vi "thickness main.vi"() -> ()   [LabVIEW 2014]
uses:
  <vilib>/userdefined/High Color/IMAQdx.ctl
  <vilib>/vision/driver/NI_Vision_Acquisition_Software.lvlib
  <vilib>/vision/NI_Vision_Development_Module.lvlib
  <vilib>/Analysis/NI_AALBase.lvlib
  <vilib>/ptbypt/NI_PtbyPt.lvlib
panel:
  in  "탭 컨트롤":enum32{"두께 측정", "vision set", "공정능력"}(tab)
  in  "두께보정":sgl=0.008
  in  "측정속도(sec)":i8
  in  "Camera Name 2":T1="cam0"
  out "Image Out":T2(plugin-control)
  out "mm":sgl
  out "Image 2":T2(plugin-control)
  out "웨이브폼 차트 3":sgl(graph)
  in  "정지 3":bool
  out "Cpk":dbl(graph)
  in  "하한규격":dbl=1.7 format="%_3f"
  in  "상한규격":dbl=1.8 format="%_3f"
  in  "측정":T3={"Contrast"=1, "Filter width"=11, "Steepness"=0, "Subsampling Ratio"=100, "Show Search Area"=TRUE, "Show Search Lines"=TRUE, "Show Edges Found"=TRUE, "Show Result"=TRUE}
  in  "입자 수":i32=20
  in  "Blue or Luma or Val or Inten":cluster{"Lower value":i32, "Upper value":i32}={"Lower value"=0, "Upper value"=93}
  in  "Green or Sat":cluster{"Lower value":i32, "Upper value":i32}={"Lower value"=0, "Upper value"=179}
  in  "Red or Hue":cluster{"Lower value":i32, "Upper value":i32}={"Lower value"=0, "Upper value"=246}
  out "Image Out 2":T2(plugin-control)
  out "Histogram":T4(graph)
  out "mm":dbl
  in  "intervals":i32=20
  out "Cpk":dbl format="%#_3g"
  out "Minimum":dbl format="%_3g"
  out "Maximum":dbl format="%#_3g"
  out "Standard Dev":dbl format="%#_3g"
  out "mean":dbl format="%.3f"
  # "칼러필터"
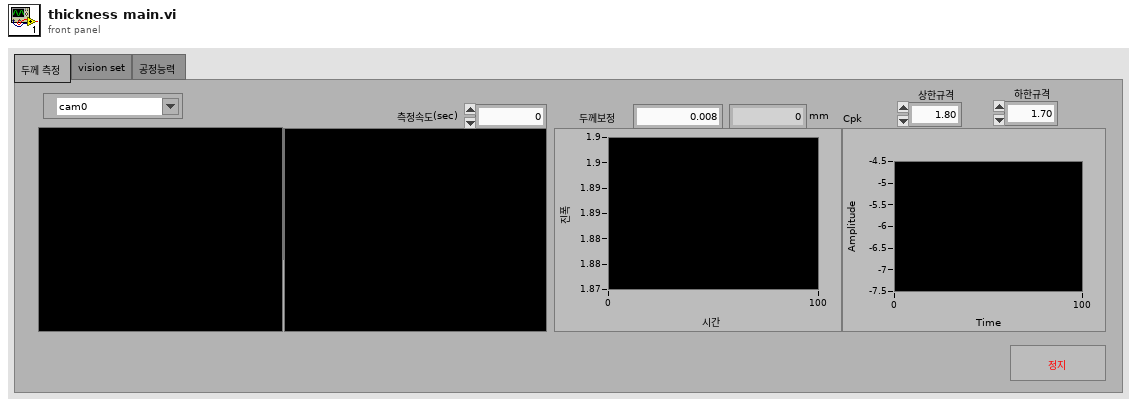
[diagram p1: front panel]
types:
  T1 = typedef "IMAQdx.ctl" = refnum<k21>
  T2 = typedef "IMAQ Image.ctl" = refnum<image>
  T3 = cluster{"Contrast":i32, "Filter width":i32, "Steepness":i32, "Subsampling Ratio":u32, "Show Search Area":bool, "Show Search Lines":bool, "Show Edges Found":bool, "Show Result":bool}
  T4 = cluster{"X Values":dbl[], "Histogram: h(x)":i32[]}
  T5 = cluster{"Global Rectangle":i32[], "Contours":cluster{"ID":enum32{"External", "Internal"}, "Type":u32, "Coordinates":i32[]}[]}
  T6 = cluster{"mm":sgl, "mm":sgl, "mm":sgl, "mm":sgl, "mm":sgl, "mm":sgl, "mm":sgl, "mm":sgl, "mm":sgl, "mm":sgl, "mm":sgl, "mm":sgl, "mm":sgl, "mm":sgl, "mm":sgl, "mm":sgl, "mm":sgl, "mm":sgl, "mm":sgl, "mm":sgl, "mm":sgl}
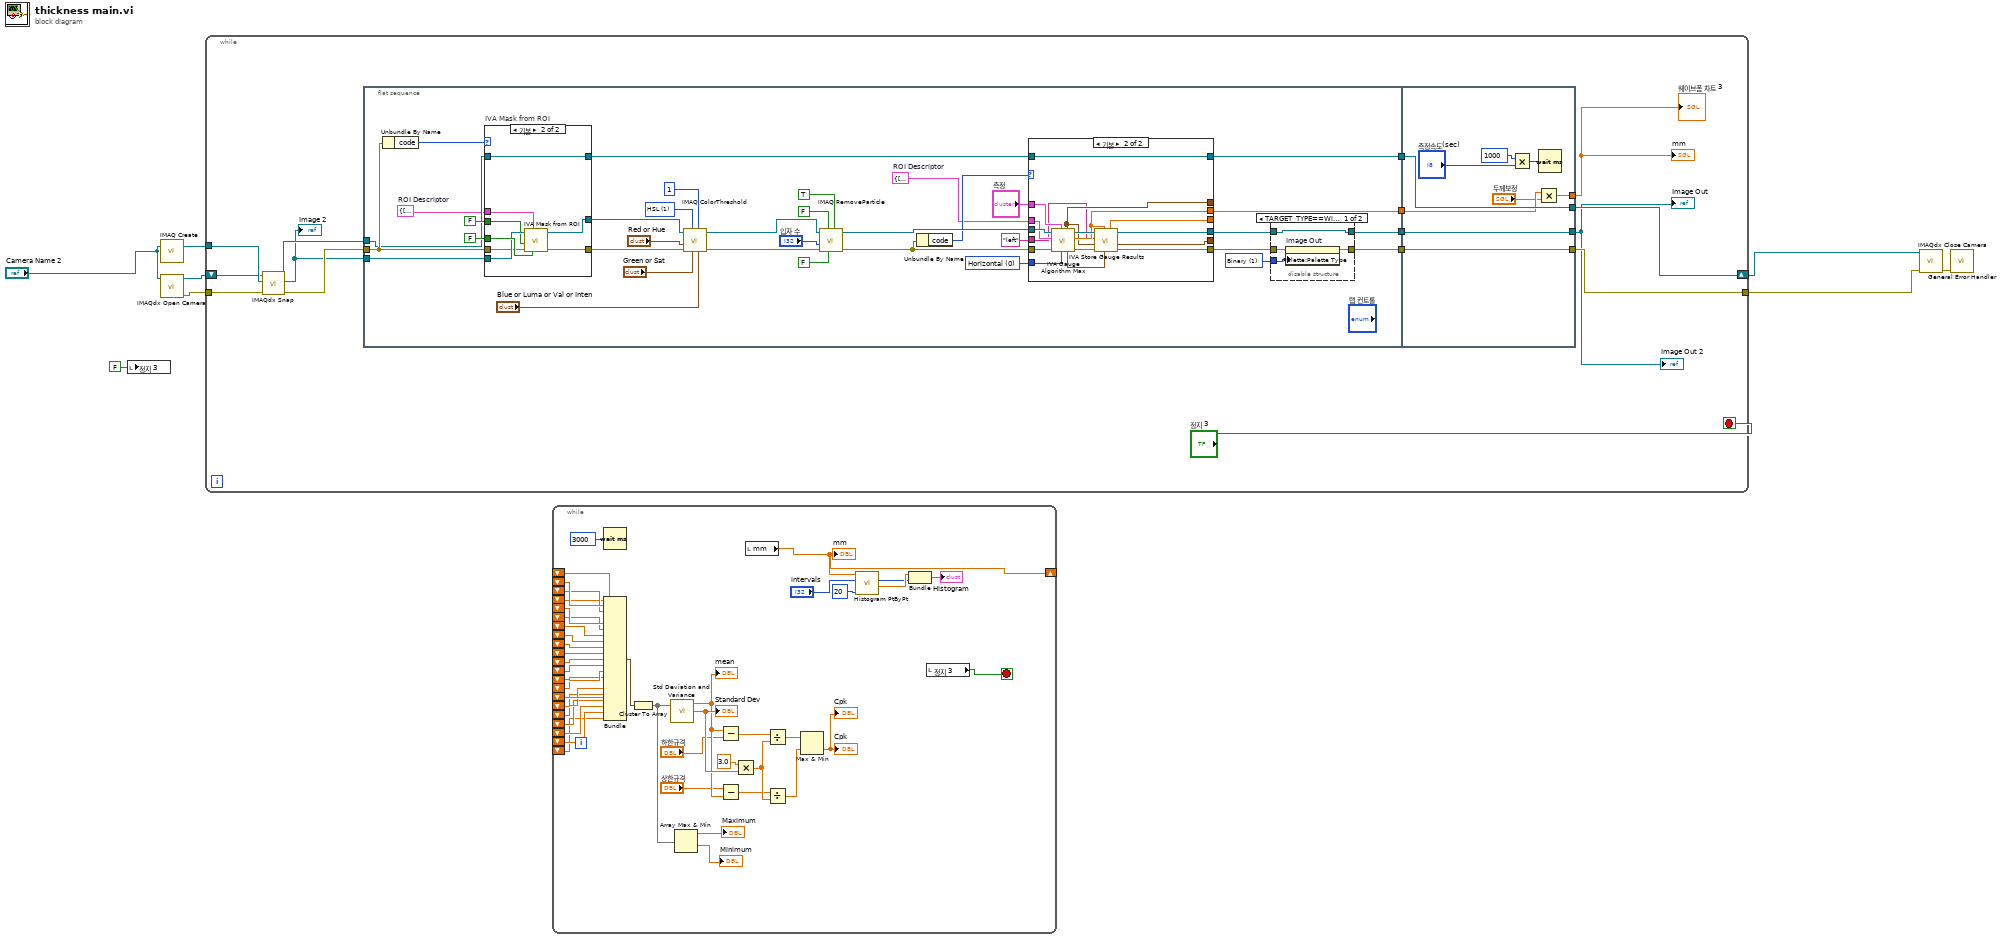
[diagram p0: block diagram]
diagram:
  n1 = local write "정지 3"(FALSE ("정지 3")) -> ()
  n2 = call "IMAQ Create"("Image Name"="Camera Name 2") -> ("New Image"=w4:T2)  [unwired: 3 in, 2 out]
  n3 = call <vilib>:"IMAQdx Open Camera.vi"("Session In"="Camera Name 2") -> ("error out"=w2:errorcluster, "Session Out"=w3:T1)  [unwired: 2 in, 7 out]
  n4 = while {
    tunnel: [w22] -> w6
    shift-right: [w19] -> w7
    shift-left: w3 -> [w11]
    tunnel: w4 -> [w12]
    tunnel: w2 -> [w10]
    stop <- "정지 3" stop-if-true
    n5 = call <vilib>:"IMAQdx Snap.vi"("error in"=w10, "Image In"=w12, "Session In"=w11) -> ("error out"=w23:errorcluster, "Image Out"=w18:T2, "Session Out"=w20:T1)  [unwired: 6 out]
    "Image 2" <- w18
    n6 = flat-sequence {
      tunnel: w23 -> [w32]
      tunnel: w18 -> [w31]
      tunnel: w20 -> [w27]
      tunnel: [w34] -> w17
      tunnel: [w30] -> w16
      tunnel: [w29] -> w15
      tunnel: [w26] -> w14
      tunnel: [w99] -> w19
      tunnel: [w94] -> w13
      tunnel: [w100] -> w22
      tunnel: [w101] -> w9
      tunnel: w17 -> [w101]
      tunnel: w16 -> [w100]
      tunnel: w15 -> [w95]
      tunnel: w14 -> [w99]
      frame #0 {
        w24 = T5 {"Global Rectangle"=[10, 36, 621, 445], "Contours"=[{"ID"=enum."External", "Type"=3, "Coordinates"=[10, 36, 621, 445]}]}  # ROI Descriptor
        w25 = T5 {"Global Rectangle"=[39, 71, 581, 408], "Contours"=[{"ID"=enum."External", "Type"=12, "Coordinates"=[39, 71, 581, 408, 0]}]}  # ROI Descriptor
        w33 = u32 1 items=["Grayscale", "Binary", "Gradient", "Rainbow", "Temperature", "User Defined"] ("Palette")
        w39 = u32 0 items=["Horizontal", "Vertical"] ("Scanning axis")
        w53 = u16 1 items=["RGB", "HSL", "HSV", "HSI"] ("Color Mode")
        n7 = Unbundle By Name(w32) -> ("code"=w55:i32)
        n8 = case "IVA Mask from ROI" shown="기본" w55 {
          tunnel: w24 -> [_ w74]
          tunnel: FALSE ("Shrink") -> [_ w73]
          tunnel: w31 -> [w66 w72]
          tunnel: w32 -> [_ w71]
          tunnel: [_ w70] -> w57
          tunnel: [w66 w69] -> w49
          tunnel: FALSE ("Out / In") -> [_ w68]
          tunnel: [w65 w67] -> w28
          tunnel: w27 -> [w65 w67]
          frame -1074396199, -1074396198 {
            # "Discard\nCoordinate\nSystem\nError"
          }
          frame Default {
            n9 = call <vilib>:"IVA Mask from ROI.vi"("Shrink"=w73, "ROI Descriptor"=w74, "error in (no error)"=w71, "Out / In"=w68, "Image Src"=w72) -> ("error out"=w70:errorcluster, "Image Out"=w69:T2)  [unwired: 5 out]
          }
        }
        n10 = call "IMAQ ColorThreshold"("Blue or Luma or Val or Inten Range"="Blue or Luma or Val or Inten", "Replace Value"=1, "Green or Sat Range"="Green or Sat", "Color Mode"=w53, "error in (no error)"=w57, "Red or Hue Range"="Red or Hue", "Image Src"=w49) -> ("error out"=w48:errorcluster, "Image Dst Out"=w43:T2)  [unwired: 1 in, 2 out]
        n11 = call "IMAQ RemoveParticle"("Connectivity 4/8 (8)"=TRUE, "Low Pass/High Pass (Low)"=FALSE, "Square/Hexa (Square)"=FALSE, "error in (no error)"=w48, "Number of Erosion"="입자 수", "Image Src"=w43) -> ("error out"=w42:errorcluster, "Image Dst Out"=w41:T2)  [unwired: 1 in, 3 out]
        n12 = Unbundle By Name(w42) -> ("code"=w37:i32)
        n13 = case "케이스 구조" shown="기본" w37 {
          tunnel: w41 -> [w76 w92]
          tunnel: w42 -> [_ w91]
          tunnel: "측정" -> [_ w90]
          tunnel: w39 -> [_ w89]
          tunnel: w25 -> [_ w88]
          tunnel: [w76 w86] -> w35
          tunnel: [_ w84] -> w38
          tunnel: [_ w83] -> w29
          tunnel: [_ w82] -> _
          tunnel: [_ w81] -> _
          tunnel: [_ w80] -> _
          tunnel: "left" ("Step Name") -> [_ w79]
          tunnel: w28 -> [w75 w77]
          tunnel: [w75 w77] -> w26
          frame -1074396199, -1074396198 {
            # "Discard Coordinate System Error"
          }
          frame Default {
            n14 = call <vilib>:"IVA Gauge Algorithm Max.vi"("Scanning axis"=w89, "Settings"=w90, "error in (no error)"=w91, "ROI Descriptor"=w88, "Image"=w92) -> ("error out"=w85:errorcluster, "Distance"=w83:sgl, "Image Out"=w87:T2, "Distance Points"=w78:cluster{"X":sgl, "Y":sgl}[], "Points of Contact"=w82:cluster{"X":sgl, "Y":sgl}[])  [unwired: 1 in, 1 out]
            n15 = call <vilib>:"IVA Store Gauge Results.vi"("Distance Points"=w78, "Distance"=w83, "error in (no error)"=w85, "Points of Contact"=w82, "Step Name"=w79, "Image in"=w87) -> ("error out"=w84:errorcluster, "Points of Contact (calibrated)"=w80:cluster{"X":sgl, "Y":sgl}[], "Image dup"=w86:T2, "Distance (calibrated)"=w81:sgl)  [unwired: 2 out]
          }
        }
        n16 = disable-structure "조건적 비활성화 구조" shown="TARGET_TYPE==Windows" {
          disable-tunnel: w38 -> [w62 w63]
          disable-tunnel: [w61 w63] -> w30
          disable-tunnel: w35 -> [w60 w64]
          disable-tunnel: [w60 w64] -> w34
          disable-tunnel: w33 -> [w59 _]
          frame condition #0 (active) {
            n17 = property on="Image Out" class="ImageControl"(error in=w62, "Palette:Palette Type"=w59) -> (error out=w61:errorcluster)  [unwired: 1 in, 1 out]
          }
          frame condition #1 {
          }
        }
      }
      frame #1 {
        n18 = Multiply(x=u32 1000 ("대기 시간(ms)"), y="측정속도(sec)") -> (x*y=w96:u32)
        n19 = Multiply(x=w95, y="두께보정") -> (x*y=w94:sgl)
        n20 = Wait (ms)(milliseconds to wait=w96) -> ()  [unwired: 1 out]
      }
    }
    "Image Out" <- w9
    "mm" <- w13
    "웨이브폼 차트 3" <- w13
    "Image Out 2" <- w9
  }
  n21 = while {
    shift-right: [w103] -> _
    shift-left: _ -> [w145]
    shift-left: _ -> [w144]
    shift-left: _ -> [w143]
    shift-left: _ -> [w142]
    shift-left: _ -> [w141]
    shift-left: _ -> [w138]
    shift-left: _ -> [w137]
    shift-left: _ -> [w136]
    shift-left: _ -> [w135]
    shift-left: _ -> [w134]
    shift-left: _ -> [w133]
    shift-left: _ -> [w132]
    shift-left: _ -> [w131]
    shift-left: _ -> [w130]
    shift-left: _ -> [w129]
    shift-left: _ -> [w128]
    shift-left: _ -> [w127]
    shift-left: _ -> [w126]
    shift-left: _ -> [w125]
    shift-left: _ -> [w107]
    shift-left: _ -> [w106]
    stop <- w102 stop-if-true
    n22 = Wait (ms)(milliseconds to wait=u32 3000) -> ()  [unwired: 1 out]
    n23 = Bundle("mm"=w145, "mm"=w144, "mm"=w143, "mm"=w142, "mm"=w141, "mm"=w138, "mm"=w137, "mm"=w136, "mm"=w135, "mm"=w134, "mm"=w133, "mm"=w132, "mm"=w131, "mm"=w130, "mm"=w129, "mm"=w128, "mm"=w127, "mm"=w126, "mm"=w125, "mm"=w107, "mm"=w106) -> (w140:T6)  [unwired: 1 in]
    n24 = Cluster To Array(cluster=w140) -> (array=w112:sgl[])
    n25 = call <vilib>:"Std Deviation and Variance.vi"("X"=w112) -> ("mean"=w120:dbl, "standard deviation"=w121:dbl)  [unwired: 1 in, 1 out]
    "mean" <- w120
    "Standard Dev" <- w121
    n26 = Array Max & Min(array=w112) -> (max value=→"Maximum":sgl, min value=→"Minimum":sgl)  [unwired: 2 out]
    n27 = Subtract(x=w120, y="하한규격") -> (x-y=w118:dbl)
    n28 = Subtract(x="상한규격", y=w120) -> (x-y=w114:dbl)
    n29 = Multiply(x=3.0, y=w121) -> (x*y=w116:dbl)
    n30 = local read "mm"() -> (w103:sgl)
    "mm" <- w103
    n31 = Divide(x=w118, y=w116) -> (x/y=w123:dbl)
    n32 = Divide(x=w114, y=w116) -> (x/y=w124:dbl)
    n33 = Max & Min(x=w123, y=w124) -> (min(x,y)=→"Cpk" →"Cpk":dbl)  [unwired: 1 out]
    n34 = call <vilib>:"Histogram PtByPt.vi"("sample length"=20, "intervals"="intervals", "x"=w103) -> ("X Values"=w109:dbl[], "Histogram: h(x)"=w108:i32[])  [unwired: 5 in, 2 out]
    n35 = Bundle("X Values"=w109, "Histogram: h(x)"=w108) -> (→"Histogram":T4)  [unwired: 1 in]
    n36 = local read "정지 3"() -> (w102:bool)
  }
  n37 = call <vilib>:"IMAQdx Close Camera.vi"("error in"=w6, "Session In"=w7) -> ("error out"=w8:errorcluster)  [unwired: 9 out]
  n38 = call <vilib>:"General Error Handler.vi"("error in (no error)"=w8) -> ()  [unwired: 2 in, 13 out]
